vi "Utilization Report.vi"   [LabVIEW 2014]
uses:
  <vilib>/Utility/error.llb/DialogType.ctl
  <vilib>/Wiresmith Technology/LabVIEW CLI/CLI Class/CLI.lvclass
types:
  T1 = cluster{"mean":dbl, "standard deviation":dbl, "99 percentile":dbl}
  T2 = cluster{"mean":dbl, "std dev":dbl, "99 percentile":dbl, "slope":dbl}
  T3 = cluster{"build_number":i32, "test_name":string, "cpu load stats":cluster{"mean":dbl, "standard deviation":dbl, "99 percentile":dbl}, "memory stats":cluster{"mean":dbl, "std dev":dbl, "99 percentile":dbl, "slope":dbl}, "size(s)":i32}
  T4 = typedef "DialogType.ctl" = u16
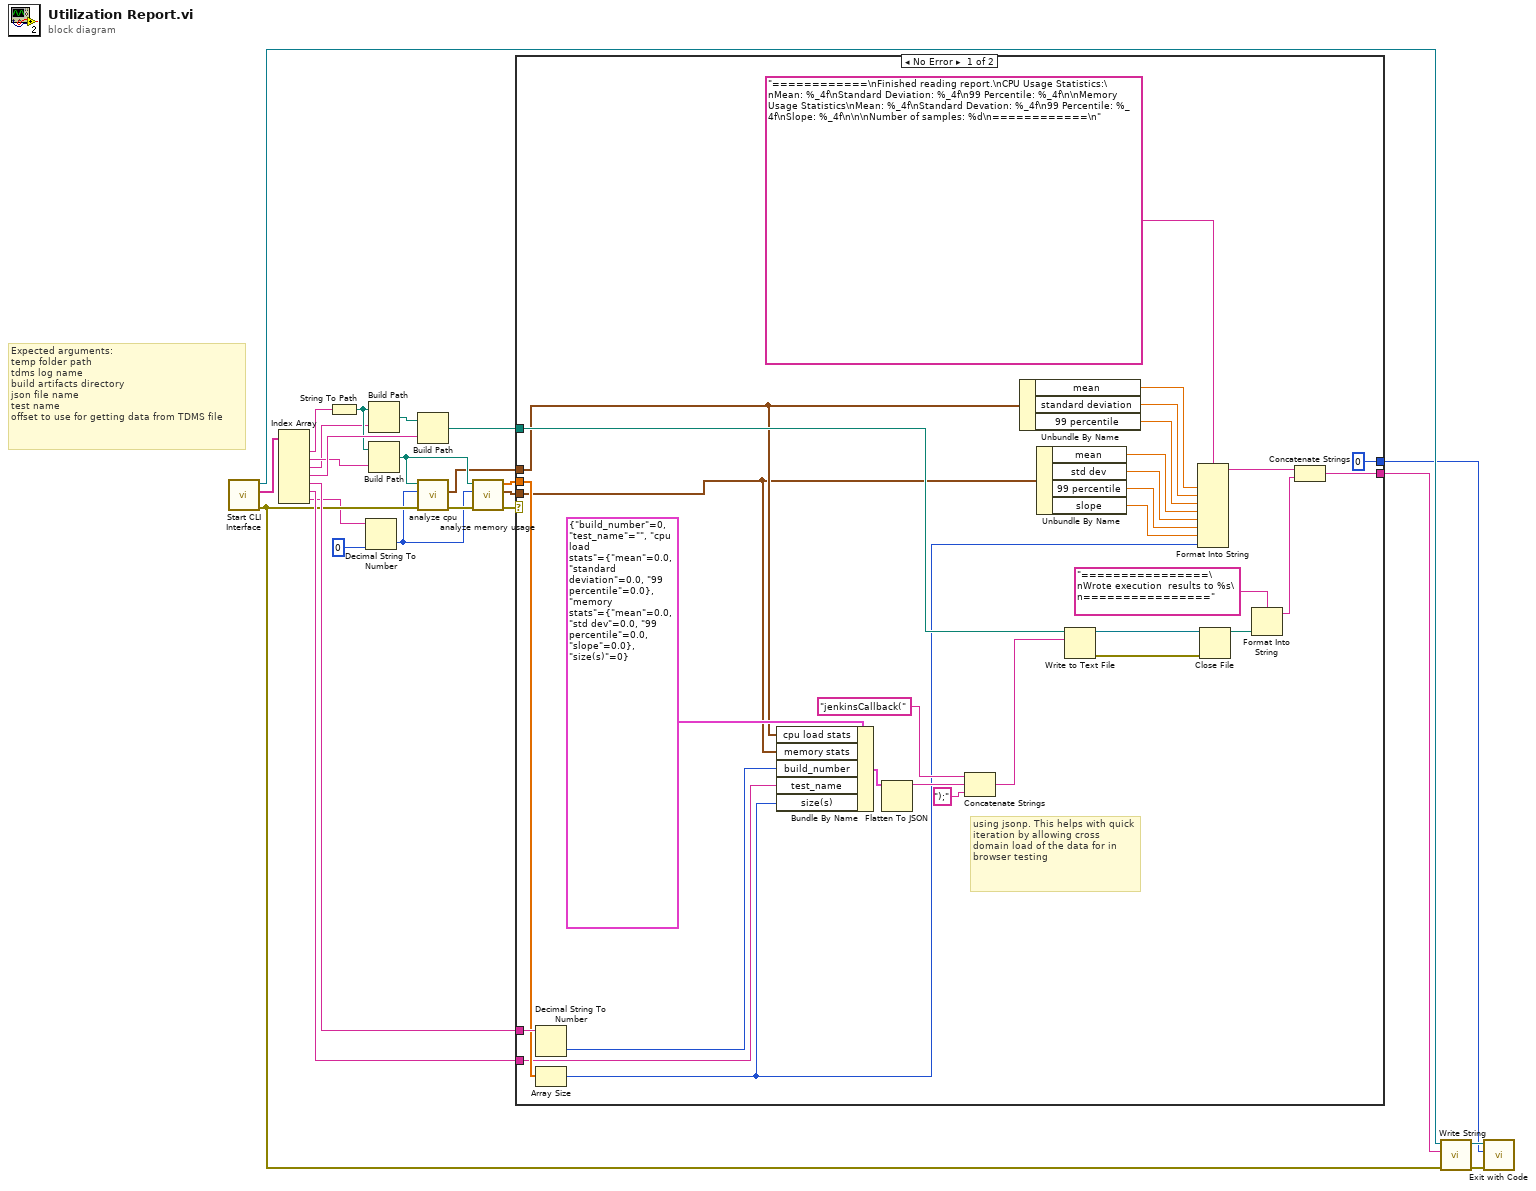
[diagram p0: block diagram]
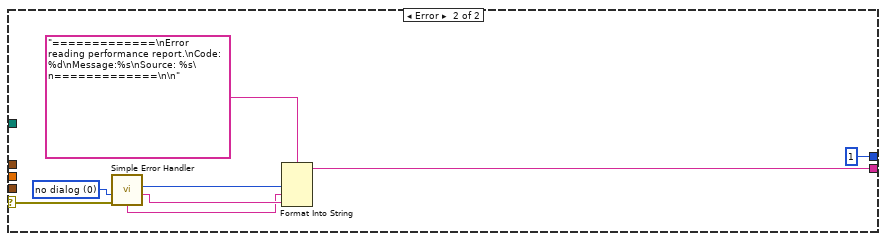
[diagram p2: hidden frame]
diagram:
  # "Expected arguments:\ntemp folder path\ntdms log name\nbuild artifacts directory\njson file name\ntest name\noffset to use for getting data from TDMS file"
  n1 = call <vilib>:"Start CLI Interface.vi"() -> ("error out"=w8:errorcluster, "Custom Parameters"=w25:string[], "CLI out"=w20:refnum<class "CLI.lvclass">)  [unwired: 9 in]
  n2 = Index Array(array=w25) -> (element #1=w24:string, element #2=w14:string, element #3=w13:string, element #4=w18:string, element #5=w12:string, element #6=w11:string, element #7=w3:string)  [unwired: 7 in]
  n3 = String To Path(string=w24) -> (path=w15:path)
  n4 = Decimal String To Number(string=w3, default (0L)=i64 0 ("offset (0)")) -> (number=w2:i64)  [unwired: 1 in, 1 out]
  n5 = Build Path(base path=w15, name or relative path=w13) -> (appended path=w16:path)
  n6 = Build Path(base path=w15, name or relative path=w14) -> (appended path=w9:path)
  n7 = Build Path(base path=w16, name or relative path=w18) -> (appended path=w17:path)
  n8 = call "analyze cpu.vi"("error in (no error)"=w8, "offset (0)"=w2, "file path"=w9) -> ("error out"=w10:errorcluster, "cpu load stats"=w7:T1)  [unwired: 6 in, 1 out]
  n9 = call "analyze memory usage.vi"("error in (no error)"=w10, "offset (0)"=w2, "file path"=w9) -> ("error out"=w4:errorcluster, "memory stats"=w6:T2, "Data"=w5:dbl[])  [unwired: 6 in]
  n10 = case shown="No Error" w4 {
    selector: w4 -> [_ w60]
    tunnel: [w37 w56] -> w21
    tunnel: [0 ("Exit Code (0)") 1 ("Exit Code (0)")] -> w19
    tunnel: w17 -> [w36 _]
    tunnel: w12 -> [w54 _]
    tunnel: w11 -> [w29 _]
    tunnel: w7 -> [w27 _]
    tunnel: w6 -> [w26 _]
    tunnel: w5 -> [w35 _]
    frame No Error {
      # "using jsonp. This helps with quick iteration by allowing cross domain load of the data for in browser testing"
      n11 = Decimal String To Number(string=w54) -> (number=w30:i32)  [unwired: 2 in, 1 out]
      n12 = Array Size(array=w35) -> (size(s)=w28:i32)
      n13 = Bundle By Name(cluster=T3 {"build_number"=0, "test_name"="", "cpu load stats"={"mean"=0.0, "standard deviation"=0.0, "99 percentile"=0.0}, "memory stats"={"mean"=0.0, "std dev"=0.0, "99 percentile"=0.0, "slope"=0.0}, "size(s)"=0}, "cpu load stats"=w27, "memory stats"=w26, "build_number"=w30, "test_name"=w29, "size(s)"=w28) -> (w50:T3)
      n14 = Flatten To JSON(anything=w50) -> (JSON string=w48:string)  [unwired: 2 in, 1 out]
      n15 = Concatenate Strings("jenkinsCallback(" ("string"), w48, ");" ("string")) -> (w47:string)
      n16 = Unbundle By Name(w27) -> ("mean"=w39:dbl, "standard deviation"=w40:dbl, "99 percentile"=w41:dbl)
      n17 = Unbundle By Name(w26) -> ("mean"=w34:dbl, "std dev"=w33:dbl, "99 percentile"=w32:dbl, "slope"=w31:dbl)
      n18 = Write to Text File(file (use dialog)=w36, text=w47) -> (refnum out=w45:refnum<file>, error out=w44:errorcluster)  [unwired: 2 in, 1 out]
      n19 = Format Into String(format string="============\nFinished reading report.\nCPU Usage Statistics:\nMean: %_4f\nStandard Deviation: %_4f\n99 Percentile: %_4f\n\nMemory Usage Statistics\nMean: %_4f\nStandard Devation: %_4f\n99 Percentile: %_4f\nSlope: %_4f\n\n\nNumber of samples: %d\n============\n", w39, w40, w41, w34, w33, w32, w31, w28) -> (resulting string=w51:string)  [unwired: 2 in, 1 out]
      n20 = Close File(refnum=w45, error in=w44) -> (path=w46:path)  [unwired: 1 out]
      n21 = Format Into String(format string="================\nWrote execution  results to %s\n================", w46) -> (resulting string=w43:string)  [unwired: 2 in, 1 out]
      n22 = Concatenate Strings(w51, w43) -> (w37:string)
    }
    frame Error {
      w61 = T4 0 items=["no dialog", "OK message", "continue or stop message", "OK message + warnings", "continue/stop + warnings"] ("type of dialog (OK msg:1)")
      n23 = call <vilib>:"Simple Error Handler.vi"("type of dialog (OK msg:1)"=w61, "error in (no error)"=w60) -> ("code out"=w59:i32, "source out"=w58:string, "message"=w57:string)  [unwired: 3 in, 2 out]
      n24 = Format Into String(format string="=============\nError reading performance report.\nCode: %d\nMessage:%s\nSource: %s\n=============\n\n", w59, w57, w58) -> (resulting string=w56:string)  [unwired: 2 in, 1 out]
    }
  }
  n25 = call <vilib>:"Write String.vi"("error in (no error)"=w8, "Text to Write"=w21, "CLI in"=w20) -> ("error out"=w23:errorcluster, "CLI out"=w22:refnum<class "CLI.lvclass">)  [unwired: 7 in]
  n26 = call <vilib>:"Exit with Code.vi"("error in (no error)"=w23, "Exit Code (0)"=w19, "CLI in"=w22) -> ()  [unwired: 8 in, 1 out]
